vi "Handle Activate Menu On Tree Item.vi"(8 "error in (no error)":errorcluster, 9 "Coords":T1, 10 "MenuRef":refnum<k9>, 11 "Test Executive Explorer in":refnum<class "Test Executive Explorer.lvclass">) -> (0 "error out":errorcluster, 1 "Discard?":bool, 3 "Test Executive Explorer out":refnum<class "Test Executive Explorer.lvclass">)   [LabVIEW 2019, in "Test Executive Explorer.lvclass"]
doc: "<RequiredOverrideReason>Override to creae create custom right click menus in the file explorer.</RequiredOverrideReason>"
uses:
  <vilib>/gpm_packages/@cs/Test-executive-builder/Example/Application/Test Executive Explorer/Test Executive Explorer/Test Executive Explorer.lvclass
  C:/Program Files/National Instruments/LabVIEW 2019/vi.lib/gpm_packages/@cs/file-explorer-extension/Source/File Explorer/File Explorer/File Explorer.lvclass
  <vilib>/Utility/miscctls.llb/LVPoint32TypeDef.ctl
  <vilib>/gpm_packages/@cs/file-explorer-extension/Source/File Explorer/File Explorer/File Explorer.lvclass/File Explorer.ctl
  <vilib>/gpm_packages/@cs/file-explorer-extension/Source/File Explorer/File Explorer/File Explorer.lvclass
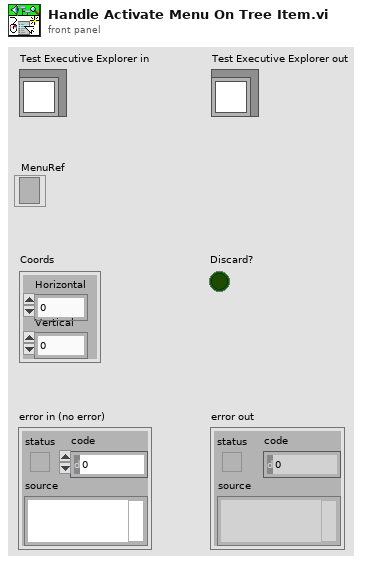
[diagram p1: front panel]
types:
  T1 = typedef "LVPoint32TypeDef.ctl" = cluster{"Horizontal":i32, "Vertical":i32}
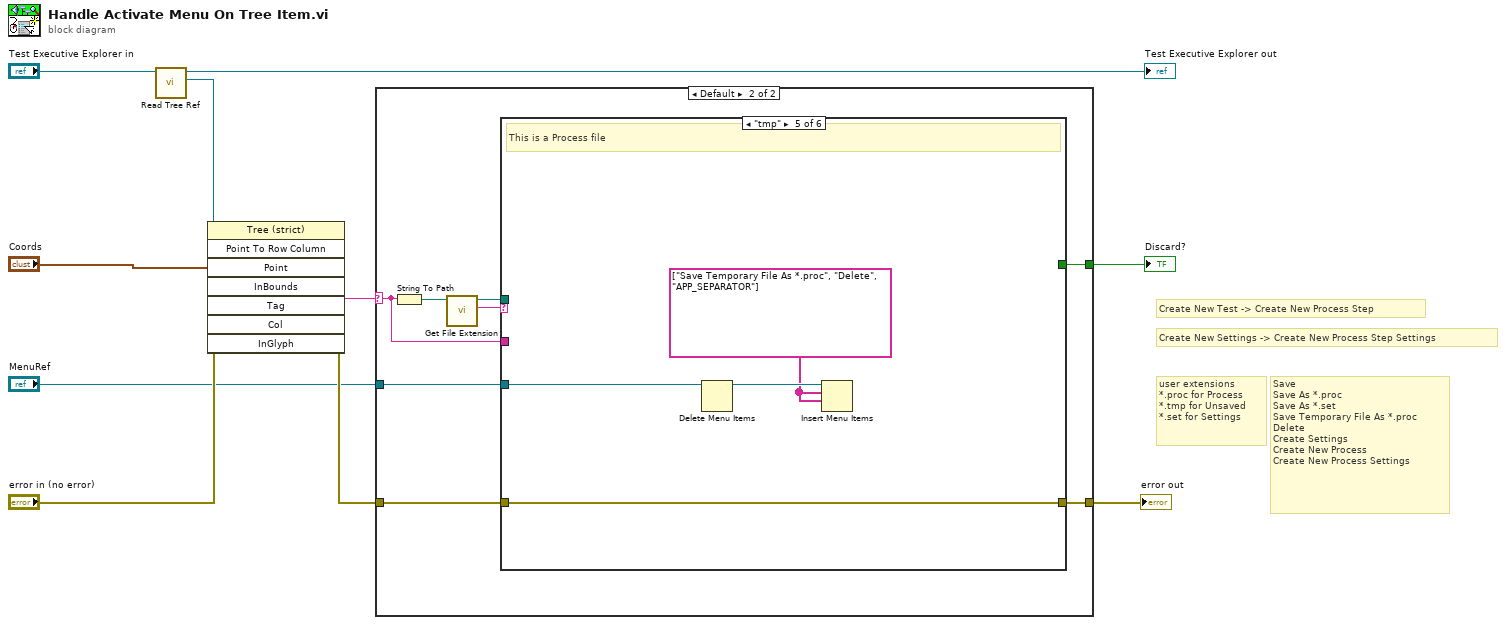
[diagram p0: block diagram]
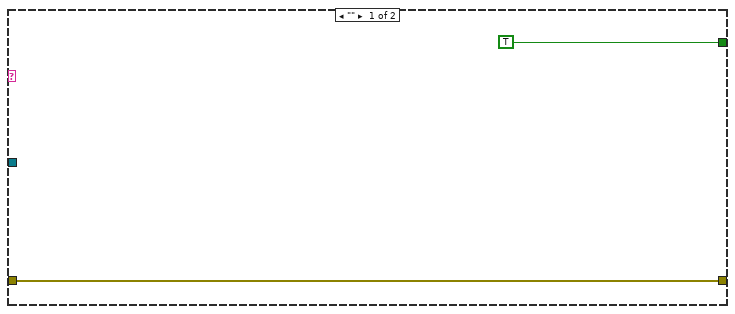
[diagram p2: hidden frame]
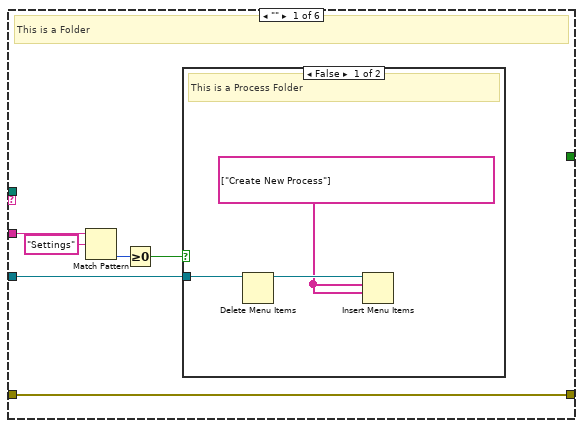
[diagram p3: hidden frame]
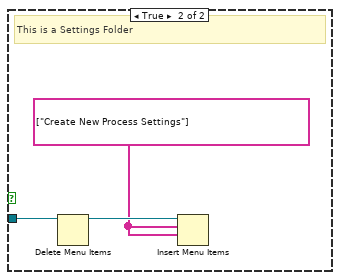
[diagram p4: hidden frame]
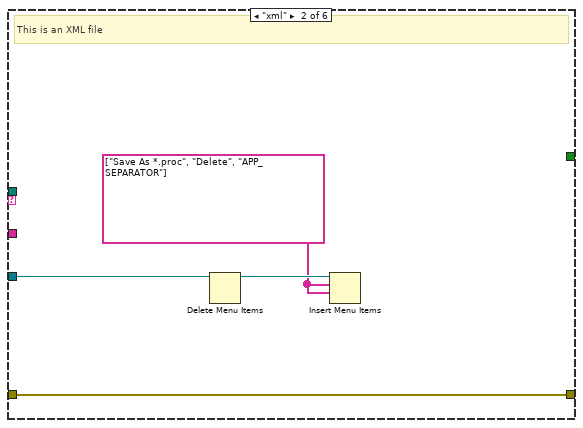
[diagram p5: hidden frame]
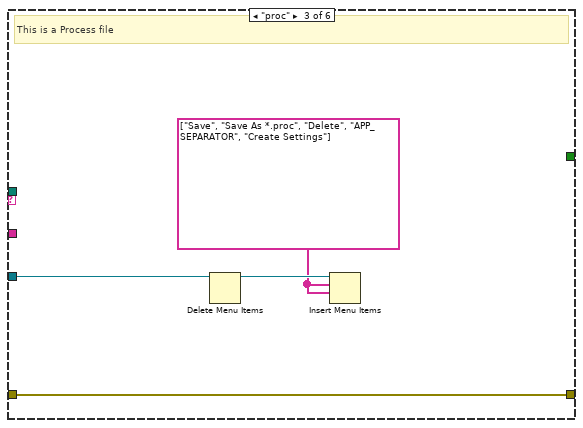
[diagram p6: hidden frame]
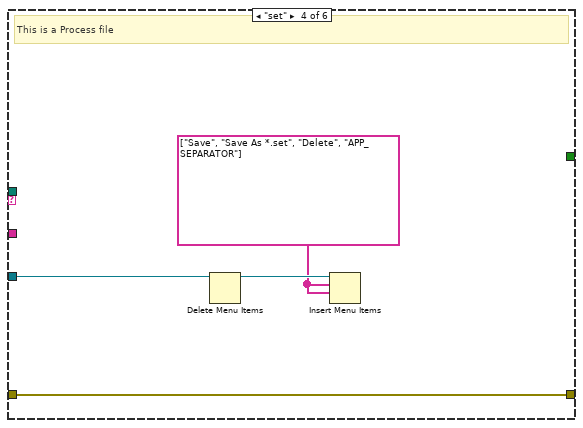
[diagram p7: hidden frame]
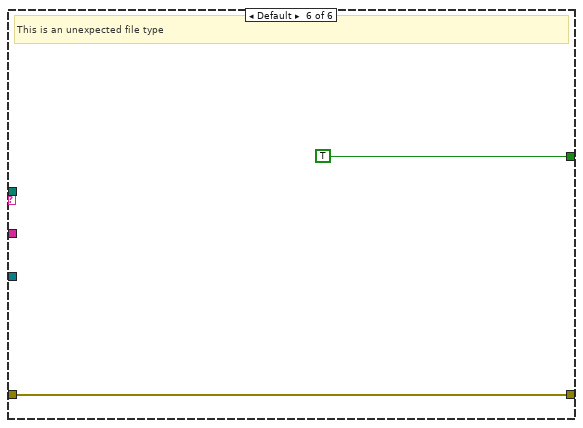
[diagram p8: hidden frame]
diagram:
  # "Save\nSave As *.proc\nSave As *.set\nSave Temporary File As *.proc\nDelete\nCreate Settings\nCreate New Process\nCreate New Process Settings"
  # "user extensions\n*.proc for Process\n*.tmp for Unsaved\n*.set for Settings"
  # "Create New Settings -> Create New Process Step Settings"
  # "Create New Test -> Create New Process Step"
  n1 = call <vilib>:"Read Tree Ref.vi"("File Explorer in"="Test Executive Explorer in") -> ("Tree Ref"=w8:refnum<vi>, "File Explorer out"=→"Test Executive Explorer out":refnum<class "Test Executive Explorer.lvclass">)  [unwired: 8 in, 1 out]
  n2 = invoke class="Tree (strict)" method="Point To Row Column"(reference=w8, error in="error in (no error)", "Point"="Coords") -> (error out=w3:errorcluster, "Tag"=w6:string)  [unwired: 5 in, 6 out]
  n3 = case shown="Default" w6 {
    selector: w6 -> [_ w13]
    tunnel: [TRUE w18] -> w4
    tunnel: w3 -> [w12 w17]
    tunnel: [w12 w16] -> w2
    tunnel: "MenuRef" -> [_ w15]
    frame "" {
    }
    frame Default {
      n4 = String To Path(string=w13) -> (path=w20:path)
      n5 = call <vilib>:"Get File Extension.vi"("file"=w20) -> ("lowercase file extension"=w19:string, "dup file"=w14:path)  [unwired: 6 in, 3 out]
      n6 = case shown="\"tmp\"" w19 {
        tunnel: [_ _ _ _ _ TRUE] -> w18
        tunnel: [w26 w36 w40 w44 w48 w49] -> w16
        tunnel: w17 -> [w26 w36 w40 w44 w48 w49]
        tunnel: w15 -> [w25 w34 w38 w42 w46 _]
        tunnel: w14 -> [_ _ _ _ _ _]
        tunnel: w13 -> [w24 _ _ _ _ _]
        frame "" {
          # "This is a Folder"
          n7 = Match Pattern(string=w24, regular expression="Settings") -> (offset past match=w22:i32)  [unwired: 1 in, 3 out]
          n8 = Greater Or Equal To 0?(x=w22) -> (x >= 0?=w21:bool)
          n9 = case shown="False" w21 {
            tunnel: w25 -> [w27 w32]
            frame False {
              w28 = string[] ["Create New Process"] ("item names")
              # "This is a Process Folder"
              n10 = Delete Menu Items(9:w27) -> (3:w29:refnum<k9>)  [unwired: 3 in, 1 out]
              n11 = Insert Menu Items(7:w28, 8:w28, 9:w29) -> ()  [unwired: 3 in, 3 out]
            }
            frame True {
              w30 = string[] ["Create New Process Settings"] ("item names")
              # "This is a Settings Folder"
              n12 = Delete Menu Items(9:w32) -> (3:w31:refnum<k9>)  [unwired: 3 in, 1 out]
              n13 = Insert Menu Items(7:w30, 8:w30, 9:w31) -> ()  [unwired: 3 in, 3 out]
            }
          }
        }
        frame "xml" {
          w33 = string[] ["Save As *.proc", "Delete", "APP_SEPARATOR"] ("item names")
          # "This is an XML file"
          n14 = Delete Menu Items(9:w34) -> (3:w35:refnum<k9>)  [unwired: 3 in, 1 out]
          n15 = Insert Menu Items(7:w33, 8:w33, 9:w35) -> ()  [unwired: 3 in, 3 out]
        }
        frame "proc" {
          w37 = string[] ["Save", "Save As *.proc", "Delete", "APP_SEPARATOR", "Create Settings"] ("item names")
          # "This is a Process file"
          n16 = Delete Menu Items(9:w38) -> (3:w39:refnum<k9>)  [unwired: 3 in, 1 out]
          n17 = Insert Menu Items(7:w37, 8:w37, 9:w39) -> ()  [unwired: 3 in, 3 out]
        }
        frame "set" {
          w41 = string[] ["Save", "Save As *.set", "Delete", "APP_SEPARATOR"] ("item names")
          # "This is a Process file"
          n18 = Delete Menu Items(9:w42) -> (3:w43:refnum<k9>)  [unwired: 3 in, 1 out]
          n19 = Insert Menu Items(7:w41, 8:w41, 9:w43) -> ()  [unwired: 3 in, 3 out]
        }
        frame "tmp" {
          w45 = string[] ["Save Temporary File As *.proc", "Delete", "APP_SEPARATOR"] ("item names")
          # "This is a Process file"
          n20 = Delete Menu Items(9:w46) -> (3:w47:refnum<k9>)  [unwired: 3 in, 1 out]
          n21 = Insert Menu Items(7:w45, 8:w45, 9:w47) -> ()  [unwired: 3 in, 3 out]
        }
        frame Default {
          # "This is an unexpected file type"
        }
      }
    }
  }
  "error out" <- w2
  "Discard?" <- w4
